vi "conv_P2T_He.vi"(6 "data_in":dbl[][](array[numeric]), 7 "He":enum16{"He4", "He3"}(ring), 8 "error in":errorcluster, 11 "P":dbl=30.0) -> (0 "error out":errorcluster, 3 "T":dbl, 4 "data_out":dbl[][](array[numeric]))   [LabVIEW 2019]
uses:
  <vilib>/Utility/file.llb/Read Delimited Spreadsheet (DBL).vi
  <vilib>/gmath/NI_Gmath.lvlib
panel:
  out "array_P":dbl[](array[numeric])
  out "array_T":dbl[](array[numeric])
  out "yi":dbl[](array[numeric]) format="%_6g"
  out "xi used":dbl[](array[numeric]) format="%_6g"
  # "VI to convert vapor pressure of He4 or He3 to temperature.\n\ndata_out can/should be fed back to data_in \nso as to read the data file only once."
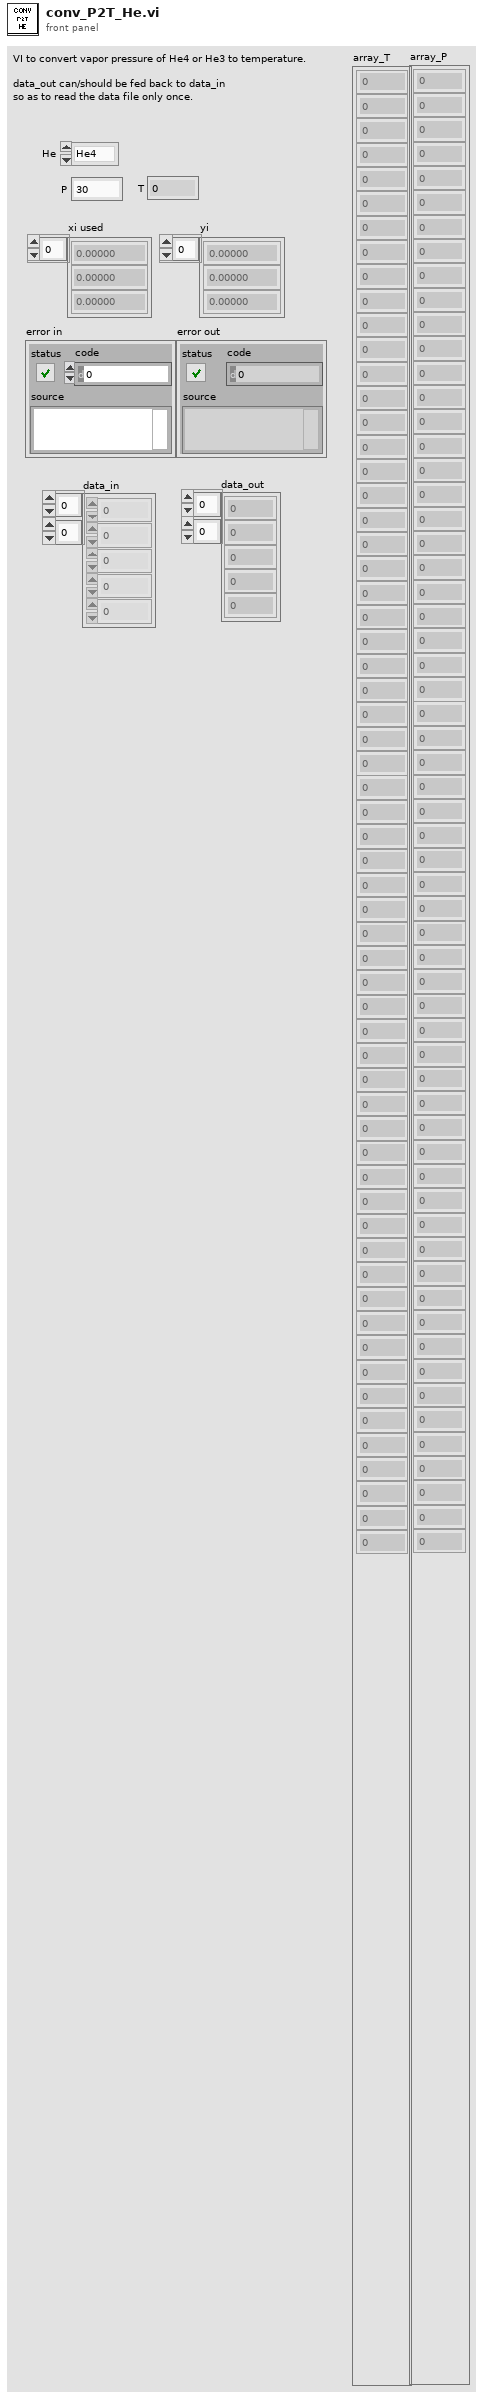
[diagram p1: front panel]
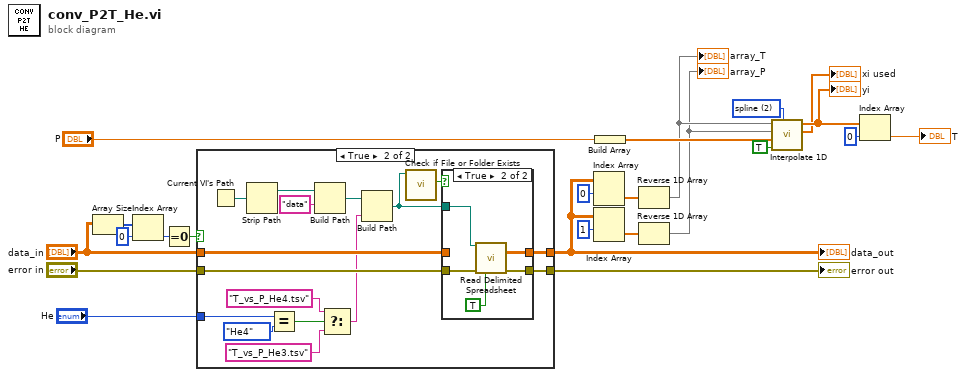
[diagram p0: block diagram]
diagram:
  w2 = 2 items=["nearest", "linear", "spline", "cubic Hermite", "Lagrange"] ("method")
  n1 = Array Size(array="data_in") -> (size(s)=w10:i32[])
  n2 = Index Array(array=w10, index=0) -> (element=w9:i32)
  n3 = Equal To 0?(x=w9) -> (x = 0?=w20:bool)
  n4 = case shown="True" w20 {
    tunnel: "error in" -> [w24 w35]
    tunnel: [w24 w34] -> w22
    tunnel: [w25 w33] -> w18
    tunnel: "data_in" -> [w25 w32]
    tunnel: "He" -> [_ w31]
    frame False {
    }
    frame True {
      n5 = Current VI's Path() -> (path=w41:path)
      n6 = Strip Path(path=w41) -> (stripped path=w40:path)  [unwired: 1 out]
      n7 = Equal?(x=w31, y=enum16{"He4", "He3"}."He4" ("He 2")) -> (x = y?=w29:bool)
      n8 = Build Path(base path=w40, name or relative path="data") -> (appended path=w38:path)
      n9 = Select(t="T_vs_P_He4.tsv" ("name or relative path"), s=w29, f="T_vs_P_He3.tsv" ("name or relative path")) -> (s? t:f=w26:string)
      n10 = Build Path(base path=w38, name or relative path=w26) -> (appended path=w36:path)
      n11 = call <vilib>:"Check if File or Folder Exists.vi"("path"=w36) -> ("file or folder exists?"=w37:bool)  [unwired: 8 in, 2 out]
      n12 = case shown="True" w37 {
        tunnel: w36 -> [_ w48]
        tunnel: w35 -> [w42 w47]
        tunnel: [w42 w46] -> w34
        tunnel: [w43 w45] -> w33
        tunnel: w32 -> [w43 _]
        frame False {
        }
        frame True {
          n13 = call-poly <vilib>:"Read Delimited Spreadsheet.vi"("file path (dialog if empty)"=w48, "error in (no error)"=w47, "transpose? (F)"=TRUE) -> ("all rows"=w45:dbl[][], "error out"=w46:errorcluster)  [unwired: 7 in, 4 out]
        }
      }
    }
  }
  "error out" <- w22
  "data_out" <- w18
  n14 = Index Array(array=w18, index (row)=0) -> (element=w7:dbl[])  [unwired: 1 in]
  n15 = Index Array(array=w18, index (row)=1) -> (element=w5:dbl[])  [unwired: 1 in]
  n16 = Build Array("P") -> (w12:dbl[])
  n17 = Reverse 1D Array(array=w7) -> (reversed array=w6:dbl[])
  "array_T" <- w6
  n18 = Reverse 1D Array(array=w5) -> (reversed array=w4:dbl[])
  "array_P" <- w4
  n19 = call <vilib>:"Interpolate 1D.vi"("method"=w2, "X is monotonic"=TRUE, "xi"=w12, "X"=w4, "Y"=w6) -> ("xi used"=→"xi used":dbl[], "yi"=w16:dbl[])  [unwired: 4 in, 1 out]
  "yi" <- w16
  n20 = Index Array(array=w16, index=0) -> (element=→"T":dbl)
